vi "4Digit File Incrementer.vi"(11 "path":path) -> (3 "appended path":path)   [LabVIEW 2014]
panel:
  out "appended path 2":path
  out "concatenated string":string
  out "name 2":string
  out "number":i32
  out "before substring 2":string
  out "name":string
  out "match substring":string
  out "before substring":string
  out "String":string
  in  "error in (no error)":errorcluster
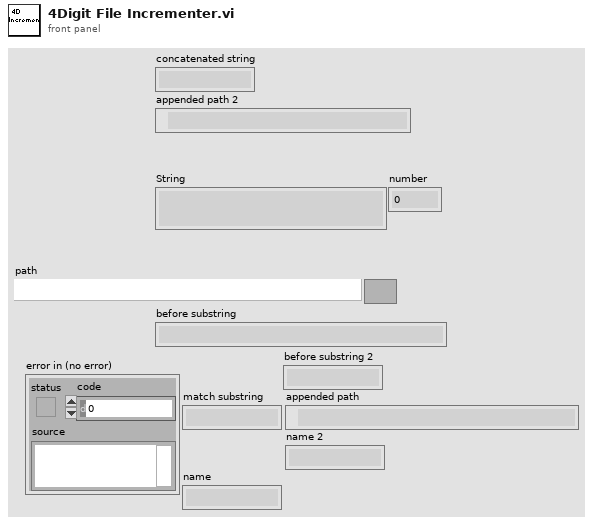
[diagram p1: front panel]
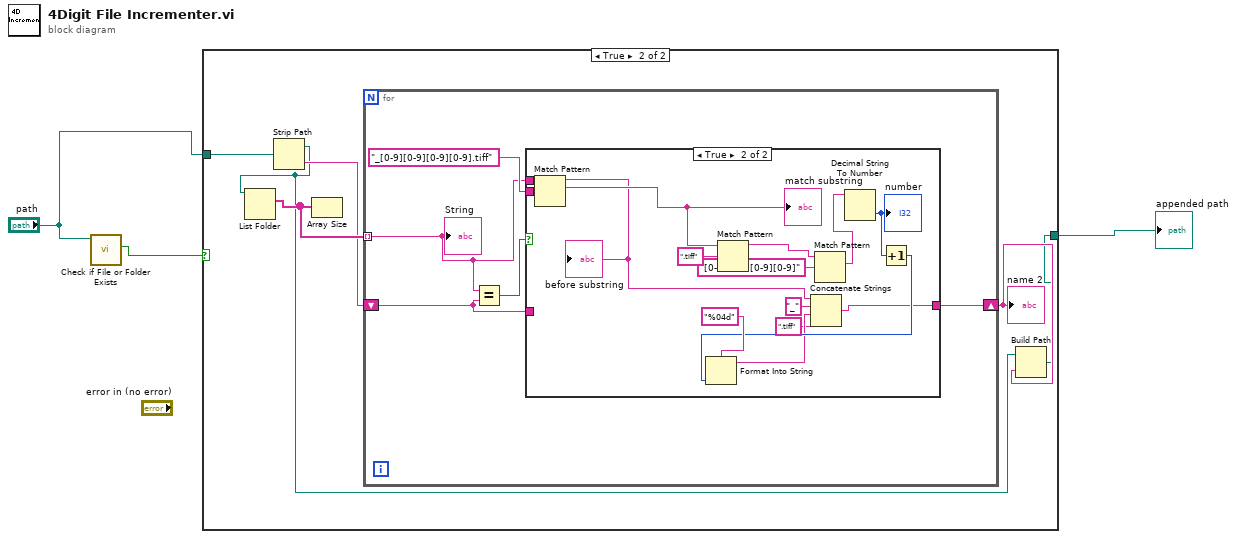
[diagram p0: block diagram]
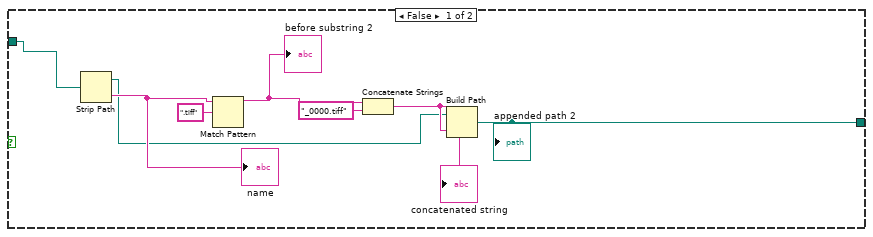
[diagram p2: hidden frame]
diagram:
  n1 = call <vilib>:"Check if File or Folder Exists.vi"("path"="path") -> ("file or folder exists?"=w2:bool)  [unwired: 8 in, 2 out]
  n2 = case shown="True" w2 {
    tunnel: "path" -> [w5 w16]
    tunnel: [w6 w12] -> w1
    frame False {
      n3 = Strip Path(path=w5) -> (stripped path=w4:path, name=w11:string)
      "name" <- w11
      n4 = Match Pattern(string=w11, regular expression=".tiff") -> (before substring=w9:string)  [unwired: 1 in, 3 out]
      "before substring 2" <- w9
      n5 = Concatenate Strings(w9, "_0000.tiff" ("string")) -> (w7:string)
      "concatenated string" <- w7
      n6 = Build Path(base path=w4, name or relative path=w7) -> (appended path=w6:path)
      "appended path 2" <- w6
    }
    frame True {
      n7 = Strip Path(path=w16) -> (stripped path=w14:path, name=w15:string)
      n8 = List Folder(path=w14) -> (filenames=w17:string[])  [unwired: 3 in, 3 out]
      n9 = Array Size(array=w17) -> ()  [unwired: 1 out]
      n10 = for {
        tunnel: w17 -> [w21] mode=indexing
        shift-right: [w19] -> w13
        shift-left: w15 -> [w18]
        n11 = Equal?(x=w21, y=w18) -> (x = y?=w20:bool)
        n12 = case shown="True" w20 {
          tunnel: w21 -> [_ w38]
          tunnel: "_[0-9][0-9][0-9][0-9].tiff" ("regular expression") -> [_ w37]
          tunnel: [w23 w27] -> w19
          tunnel: w18 -> [w23 _]
          frame False {
          }
          frame True {
            n13 = Match Pattern(string=w38, regular expression=w37) -> (before substring=w33:string, match substring=w36:string)  [unwired: 1 in, 2 out]
            "before substring" <- w33
            "match substring" <- w36
            n14 = Match Pattern(string=w36, regular expression=".tiff") -> (before substring=w26:string)  [unwired: 1 in, 3 out]
            n15 = Match Pattern(string=w26, regular expression="[0-9][0-9][0-9][0-9]") -> (match substring=w24:string)  [unwired: 1 in, 3 out]
            n16 = Decimal String To Number(string=w24) -> (number=w34:i32)  [unwired: 2 in, 1 out]
            "number" <- w34
            n17 = Increment(x=w34) -> (x+1=w31:i32)
            n18 = Format Into String(format string="%04d", w31) -> (resulting string=w29:string)  [unwired: 2 in, 1 out]
            n19 = Concatenate Strings(w33, "_" ("string"), w29, ".tiff" ("string")) -> (w27:string)
          }
        }
        "String" <- w21
      }
      "name 2" <- w13
      n20 = Build Path(base path=w14, name or relative path=w13) -> (appended path=w12:path)
    }
  }
  "appended path" <- w1
